vi "setOutputGain.vi"(8 "error in (no error)":errorcluster, 10 "OutputGain":dbl[](array[numeric]), 11 "Instrument.Lockin in":refnum<class "Instrument.Lockin.lvclass">) -> (0 "error out":errorcluster, 3 "Instrument.Lockin out":refnum<class "Instrument.Lockin.lvclass">)   [LabVIEW 2019, in "Instrument.Lockin.lvclass"]
doc: "API to put lockin into remote mode.\n\nIf address=\"\", this API reads from localhost\nIf address is remote lockin, you need to add this computer to allowed whitelist on the lockin computer you are trying to access."
uses:
  Instrument.Lockin.lvclass
  C:/Program Files (x86)/National Instruments/LabVIEW 2019/user.lib/LevyLab/Levylab Instruments/SMOs/Instrument/Instrument.lvclass
  Typedefs/API/Lockin.Commands--Enum.ctl
  <userlib>/LevyLab/Instrument Framework/SMOs/Instrument/Instrument.lvclass/Instrument.ctl
  16b0612a-153c-498e-8e8b-4591927cf31d.vi
  16b0612a-153c-498e-8e8b-4591927cf31d.vi/d69ba1d1-fd8d-4ad3-8bab-c4e383764c18.vi
  16b0612a-153c-498e-8e8b-4591927cf31d.vi/d69ba1d1-fd8d-4ad3-8bab-c4e383764c18.vi/46903cfd-925b-4e65-a4a0-6f608bee4bee.vi
  <userlib>/LevyLab/Instrument Framework/SMOs/Instrument/API/Send and Receive.vi
  16b0612a-153c-498e-8e8b-4591927cf31d.vi/d69ba1d1-fd8d-4ad3-8bab-c4e383764c18.vi/46903cfd-925b-4e65-a4a0-6f608bee4bee.vi/26a599b9-c806-4f71-b105-258e68c1b4bc.vi
  16b0612a-153c-498e-8e8b-4591927cf31d.vi/d69ba1d1-fd8d-4ad3-8bab-c4e383764c18.vi/46903cfd-925b-4e65-a4a0-6f608bee4bee.vi/bccb1efc-f299-470a-9f61-ef165fafd250.vi
  <userlib>/LevyLab/Instrument Framework/SMOs/Instrument/API/Enum to String.vi
  <userlib>/LevyLab/Instrument Framework/SMOs/RemoteControl/API/Send and Receive.vi
  <vilib>/Utility/Data Type/Get Type Information.vi
  <vilib>/JDP Science/JSONtext/JSON text to Variant.vi
  <vilib>/JDP Science/JSONtext/LVClass Serializer/JSONtext LVClass Serializer.lvclass
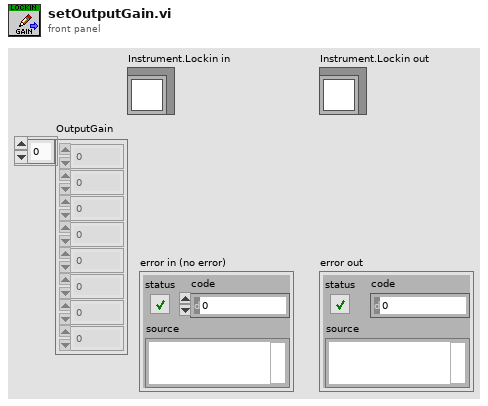
[diagram p1: front panel]
types:
  T1 = typedef "Instrument.Lockin.lvclass/Lockin.Commands--Enum.ctl" = enum16{"setAO", "setAO_Amplitude", "setAO_DC", "setAO_Frequency", "setAO_Phase", "setAO_Function", "setAO_I+", "setREF", "setREF_Frequency", "setREF_Phase", "setREF_TC", "setREF_Roll-Off", "setDAQ", "setSampling", "setOffset", "setState", "getState", "getAO", "getAI", "getResults", "getSampling", "getAOconfig", "getREFconfig", "setInputGain", "setOutputGain", "getInputGain", "getOutputGain", "setSamplingMode", "getSamplingMode", "setSweep", "getStatus", "getSweepResults", "getSweepWaveforms", "startSweep", "stopSweep", "setAUX", "getAUX", "getRefreshTime"}
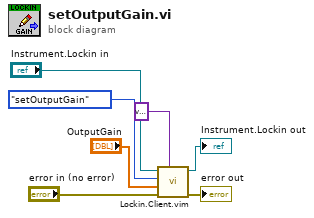
[diagram p0: block diagram]
diagram:
  n1 = call "Lockin.Client.vim"("Data Out type"=variant, "error in (no error)"="error in (no error)", "Data"="OutputGain", "Command"=Lockin.Commands--Enum."setOutputGain", "Instrument.Lockin in"="Instrument.Lockin in") -> ("error out"=→"error out":errorcluster, "Instrument.Lockin out"=→"Instrument.Lockin out":refnum<class "Instrument.Lockin.lvclass">)  [unwired: 4 in, 1 out]
